vi "Tx Inline Wait.vi"(8 "error in (no error)":errorcluster, 11 "Framework in":refnum<class "Framework.lvclass">) -> (0 "error out":errorcluster, 3 "Framework out":refnum<class "Framework.lvclass">)   [LabVIEW 2017, in "DSF Core.lvlib" / "Framework.lvclass"]
uses:
  Framework.lvclass
  Framework.lvclass/Framework.ctl
  Plugin/Plugin.lvclass/Plugin.ctl
  Timing/Timing.lvclass/Timing.ctl
  Transfer Group/Transfer Group.lvclass/Transfer Group.ctl
  Debug/Debug Flags/Debug Flags.lvclass/Debug Flags.ctl
  Debug/FIFO Flags/FIFO Flags.lvclass/FIFO Flags.ctl
  Transfer/Transfer.lvclass/Transfer.ctl
  <vilib>/NI/Memory Manager/Classes/Pointer/Memory.Pointer.lvclass/Memory.Pointer.ctl
  Transfer Group/Move Channels to Engine.vi
  Transfer Group/Get Timing.vi
  Transfer Group/Retrieve from FIFO.vi
  Plugin/Get Timing.vi
  Timing/Is Active Cycle.vi
  Transfer Group/Get Transfers.vi
  Transfer/Get Inline Buffer.vi
  Transfer/Get Intermediate Buffer.vi
  <vilib>/NI/Memory Manager/Classes/Pointer/Memory.Pointer.Copy All.vi
  Transfer Group/Read Return FIFO.vi
  Timing/Get Decimation.vi
  Timing/Get Offset.vi
  <vilib>/NI/Memory Manager/Classes/Pointer/Memory.Pointer.Get Size.vi
  <vilib>/NI/Memory Manager/Classes/Pointer/Memory.Pointer.Copy.vi
  Transfer Group/Get Return FIFO.vi
  Transfer Group/Get Debug Flags.vi
  Debug/Debug Flags/Get FIFO Flags.vi
  Debug/FIFO Flags/Get Infinite Timeouts.vi
  <vilib>/NI/Memory Manager/Classes/Pointer/Memory.Pointer.Copy.No Check.vi
  <vilib>/NI/Memory Manager/Classes/Pointer/Memory.Pointer.Parameter Check.Subset.vi
  <vilib>/NI/Memory Manager/Classes/Pointer/Memory.Pointer.Parameter Check.Null Pointer.vi
  <vilib>/NI/Memory Manager/Classes/Pointer/Memory.Pointer.Get Address.vi
  <vilib>/NI/Memory Manager/Classes/Pointer/Memory.Pointer.Errors.vi
  <vilib>/NI/Memory Manager/Classes/Pointer/Memory.Pointer.Errors.Out of Bounds.vi
  <vilib>/NI/Memory Manager/Classes/Pointer/Memory.Pointer.Errors.Null Pointer.vi
  <vilib>/NI/Memory Manager/VIs/Source.Write.String.vi
  <vilib>/NI/Memory Manager/Classes/Pointer/Memory.Pointer.Errors.Write Pointer Size.vi
  <vilib>/NI/Memory Manager/Classes/Pointer/Memory.Pointer.Errors.Create Error.vi
  <vilib>/NI/Memory Manager/VIs/Source.Write.Scalar.Base10.vi
  <vilib>/NI/Memory Manager/VIs/Source.Write.Scalar.Base10 (U64).vi
  <vilib>/NI/Memory Manager/VIs/New Error Cluster Constant.vi
  <vilib>/NI/Memory Manager/VIs/New Error Cluster Constant (512B).vi
  <vilib>/NI/Memory Manager/VIs/Error Cluster.Set Status.vi
  <vilib>/NI/Memory Manager/VIs/Error Cluster.Set Code.vi
  <vilib>/NI/Memory Manager/VIs/Error Cluster.Set VI Source.vi
  <vilib>/NI/Memory Manager/Constants/Memory.Constants.vi
  <vilib>/NI/Memory Manager/Constants/Memory.Constants.Library Name.vi
  <vilib>/NI/Memory Manager/Classes/Pointer/Memory.Pointer.Errors.Get Info.vi
  Pointer/DBL Pointer.lvclass
  C:/Program Files (x86)/National Instruments/LabVIEW 2017/vi.lib/NI/Memory Manager/Classes/Pointer/Memory.Pointer.lvclass
  Transfer Group/Errors.vi
  Transfer Group/Return Timeout Error.vi
  Plugin/Plugin.lvclass
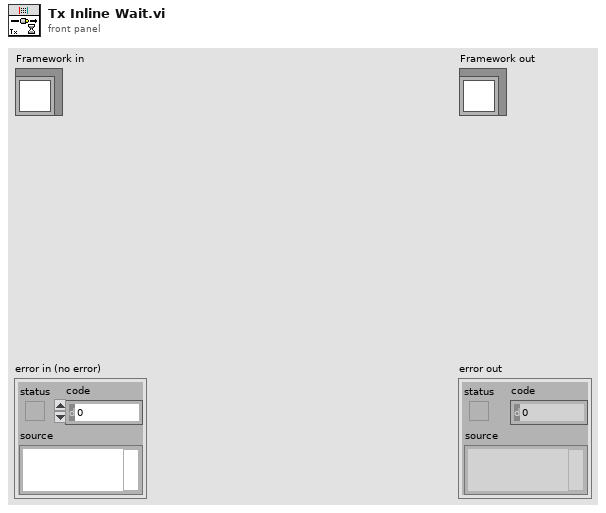
[diagram p1: front panel]
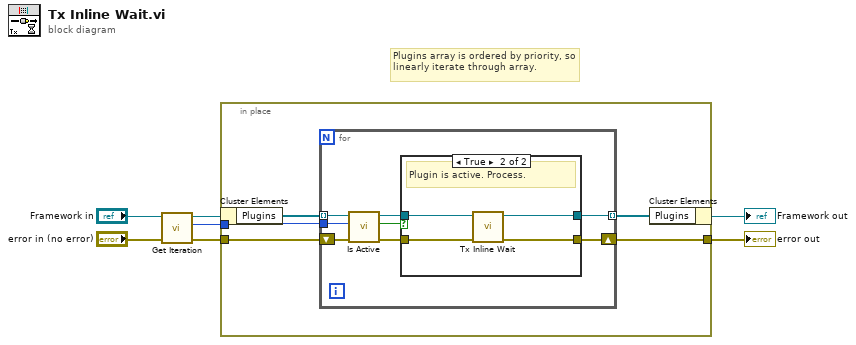
[diagram p0: block diagram]
diagram:
  # "Plugins array is ordered by priority, so linearly iterate through array."
  n1 = call "Get Iteration.vi"("Framework in"="Framework in") -> ("iteration"=w3:u64, "Framework out"=w1:refnum<class "Framework.lvclass">)  [unwired: 9 in]
  n2 = in-place {
    in-place-border: "error in (no error)" -> [w11]
    in-place-border: [w10] -> w5
    in-place-border: w3 -> [w7]
    n3 = in-place-cluster #1(w1) -> ("Plugins"=w9:refnum<class "Plugin.lvclass">[])
    n4 = for {
      tunnel: w9 -> [w16] mode=indexing
      tunnel: [w18] -> w8 mode=indexing
      shift-right: [w17] -> w10
      shift-left: w11 -> [w13]
      tunnel: w7 -> [w12]
      n5 = call "Is Active.vi"("cycle count"=w12, "Plugin in"=w16) -> ("active this cycle?"=w14:bool, "Plugin out"=w15:refnum<class "Plugin.lvclass">)  [unwired: 8 in]
      n6 = case shown="True" w14 {
        tunnel: w15 -> [w20 w24]
        tunnel: [w20 w21] -> w18
        tunnel: [w19 w22] -> w17
        tunnel: w13 -> [w19 w23]
        frame False {
          # "Plugin is not active. Skip."
        }
        frame True {
          # "Plugin is active. Process."
          n7 = call "Tx Inline Wait.vi"("error in (no error)"=w23, "Plugin in"=w24) -> ("error out"=w22:errorcluster, "Plugin out"=w21:refnum<class "Plugin.lvclass">)  [unwired: 8 in]
        }
      }
    }
    n8 = in-place-cluster #1("Plugins"=w8) -> (→"Framework out":refnum<class "Framework.lvclass">)
  }
  "error out" <- w5
